vi "Array_Investigation Part 1.vi"() -> ()   [LabVIEW 2014]
doc: "This VI is an exercise in the LabVIEW Core I course.\n\nEnter the number of columns and rows you want generated, then run the VI. This VI generates an array with the number of rows and columns you specify."
panel:
  out "Array":dbl[][](array[numeric])
  in  "Rows":i32=80
  in  "Columns":i32=80
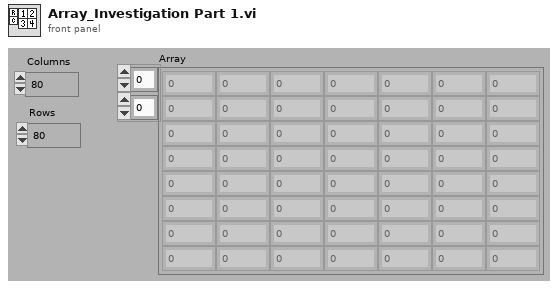
[diagram p1: front panel]
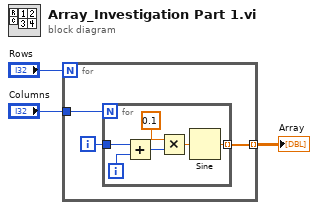
[diagram p0: block diagram]
diagram:
  n1 = for {
    N: "Rows" -> [_]
    tunnel: [w6] -> w1 mode=indexing
    tunnel: "Columns" -> [w5]
    i -> [w4]
    n2 = for {
      N: w5 -> [_]
      tunnel: [w12] -> w6 mode=indexing
      tunnel: w4 -> [w9]
      i -> [w10]
      n3 = Add(x=w9, y=w10) -> (x+y=w11:i32)
      n4 = Multiply(x=0.1, y=w11) -> (x*y=w8:dbl)
      n5 = Sine(x=w8) -> (sin(x)=w12:dbl)
    }
  }
  "Array" <- w1
